vi "CompressionDecorator_Create.vi"(8 "error in (no error)":errorcluster, 10 "Source":refnum<class "DataSource.lvclass">, 11 "reference in":refnum<class "CompressionDecorator.lvclass">) -> (0 "error out":errorcluster, 3 "reference out":refnum<class "CompressionDecorator.lvclass">)   [LabVIEW 2020, in "CompressionDecorator.lvclass"]
uses:
  CompressionDecorator.lvclass
  C:/Projects/OpenGDS_DesignPatterns/Decorator3/DataSourceDecorator_class/DataSourceDecorator.lvclass
  DataSource_interface/DataSource.lvclass
  DataSourceDecorator_class/DataSourceDecorator.lvclass
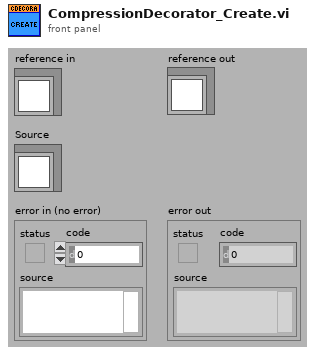
[diagram p1: front panel]
types:
  T1 = typedef "CompressionDecorator.lvclass/ObjectAttributes.ctl" = cluster{"CompLevel":i32}
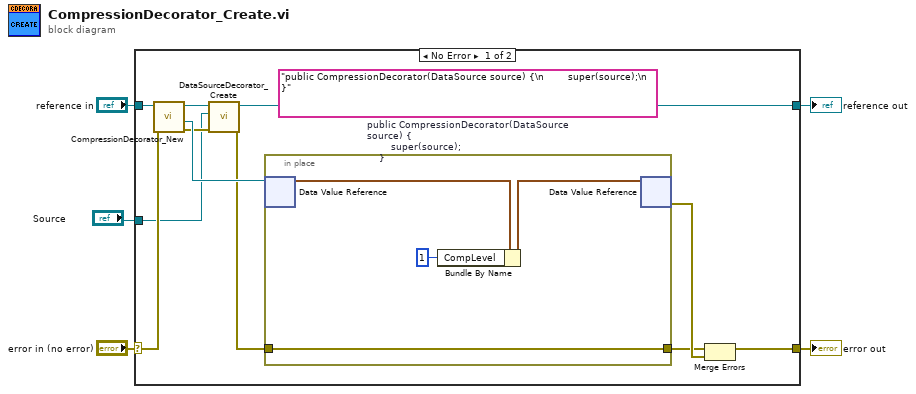
[diagram p0: block diagram]
diagram:
  n1 = case shown="No Error" "error in (no error)" {
    selector: "error in (no error)" -> [w12 w22]
    tunnel: [w10 w22] -> w4
    tunnel: "reference in" -> [w14 w21]
    tunnel: [w9 w21] -> w2
    tunnel: "Source" -> [w6 _]
    frame No Error {
      (unwired) "public CompressionDecorator(DataSource source) {\n        super(source);\n    }"  # public CompressionDecorator(DataSource source) {         super(source);     }
      n2 = call "CompressionDecorator_New.vi"("error in (no error)"=w12, "reference in"=w14) -> ("error out"=w13:errorcluster, "DVRRefOut"=w16:refnum<data-value>, "reference out"=w15:refnum<class "CompressionDecorator.lvclass">)  [unwired: 6 in, 1 out]
      n3 = call "DataSourceDecorator_Create.vi"("error in (no error)"=w13, "Source"=w6, "reference in"=w15) -> ("error out"=w8:errorcluster, "reference out"=w9:refnum<class "CompressionDecorator.lvclass">)  [unwired: 7 in]
      n4 = in-place {
        in-place-border: w8 -> [w20]
        in-place-border: [w20] -> w7
        n5 = in-place-dvr #1(w16) -> (w19:T1)  [unwired: 1 out]
        n6 = Bundle By Name(cluster=w19, "CompLevel"=1) -> (w18:T1)
        n7 = in-place-dvr #1(w18) -> (w11:errorcluster)  [unwired: 1 out]
      }
      n8 = Merge Errors(w7, w11) -> (w10:errorcluster)
    }
    frame Error {
    }
  }
  "error out" <- w4
  "reference out" <- w2
